vi "Setup.vi"(9 "Active Project":refnum<vi>, 10 "NI.LV.Dialog Instance":refnum<vi>) -> (1 "Project Type Name Library File Path":T1, 2 "Target":string, 3 "Script out":refnum<class "_Rename.lvclass">, 4 "All Type Name Library File Path":T1)   [LabVIEW 2025, in "_Rename.lvlib" / "_Rename.lvclass"]
uses:
  _Rename.lvclass
  _Shared/Type Name Library File Path.ctl
  _Shared/Type.ctl
  _Shared/Name Library File Path.ctl
  _Rename.lvclass/_Rename.ctl
  _Shared/Project Stuff/Project Stuff.lvclass
  _Shared/_Shared.lvlib
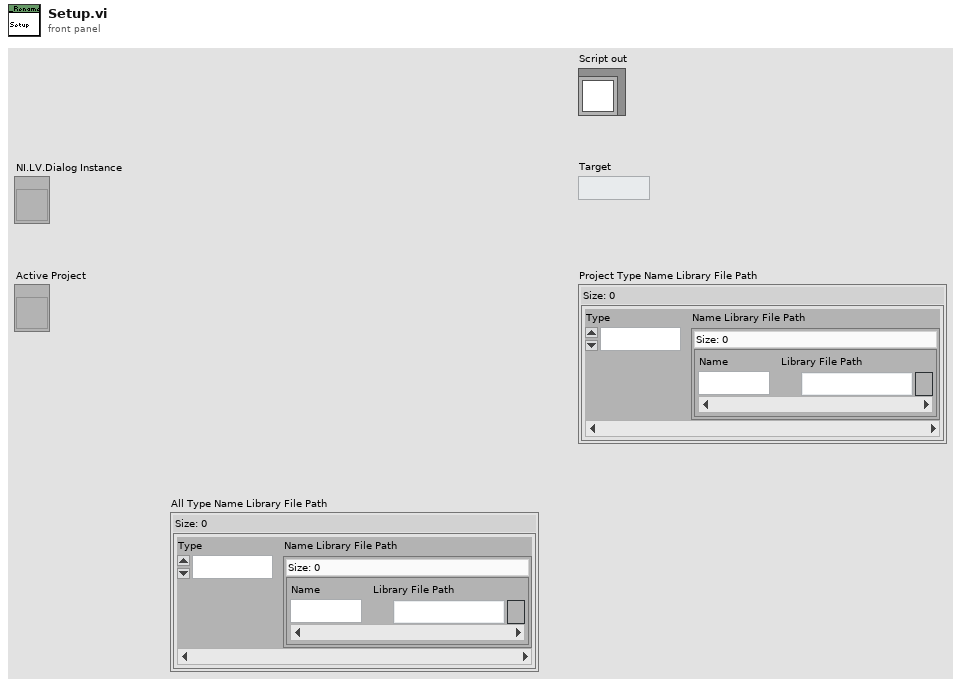
[diagram p1: front panel]
types:
  T1 = typedef "_Shared.lvlib/Type Name Library File Path.ctl" = map{T2, T3}
  T2 = typedef "_Shared.lvlib/Type.ctl" = enum16{"Actor", "Msg"}
  T3 = typedef "_Shared.lvlib/Name Library File Path.ctl" = map{string, path}
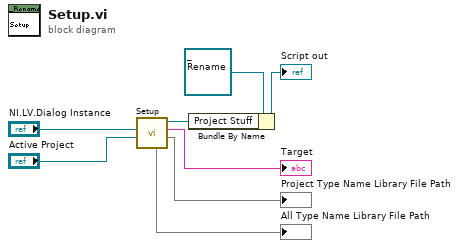
[diagram p0: block diagram]
diagram:
  n1 = call "Setup.vi"("Active Project"="Active Project", "NI.LV.Dialog Instance"="NI.LV.Dialog Instance") -> ("Project Type Name Library File Path"=→"Project Type Name Library File Path":T1, "Target"=→"Target":string, "Project Stuff out"=w6:refnum<class "Project Stuff.lvclass">, "All Type Name Library File Path"=→"All Type Name Library File Path":T1)  [unwired: 6 in]
  n2 = Bundle By Name(cluster=refnum<class "_Rename.lvclass"> refnum ("Script out"), "Project Stuff"=w6) -> (→"Script out":refnum<class "_Rename.lvclass">)
